vi "fields format list items from post.vi"(5 "Post (empty)":T1) -> (2 "List Options":string[](array[string]))   [LabVIEW 2011]
uses:
  Addons/internet/utils/keyedarr.llb/Keyed Array.ctl
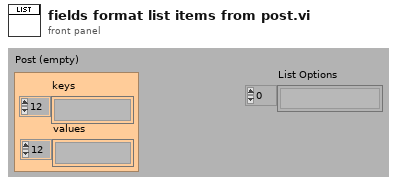
[diagram p1: front panel]
types:
  T1 = typedef "Keyed Array.ctl" = cluster{"keys":string[], "values":string[]}
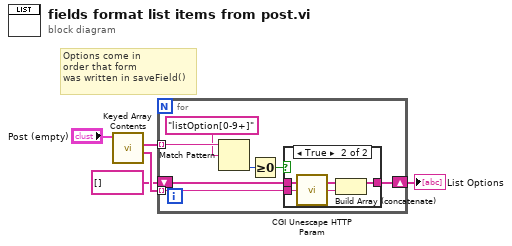
[diagram p0: block diagram]
diagram:
  # "Options come in\norder that form\nwas written in saveField()"
  n1 = call "Keyed Array Contents.vi"("array in"="Post (empty)") -> ("values"=w3:string[], "keys"=w4:string[])  [unwired: 5 out]
  n2 = for {
    tunnel: w4 -> [w12] mode=indexing
    tunnel: w3 -> [w9] mode=indexing
    shift-right: [w6] -> w1
    shift-left: string[] [] -> [w7]
    n3 = Match Pattern(string=w12, regular expression="listOption[0-9+]") -> (offset past match=w11:i32)  [unwired: 4 out]
    n4 = Greater Or Equal To 0?(x=w11) -> (x >= 0?=w8:bool)
    n5 = case shown="True" w8 {
      tunnel: w9 -> [_ w15]
      tunnel: w7 -> [w13 w17]
      tunnel: [w13 w16] -> w6
      frame False {
      }
      frame True {
        n6 = call "CGI Unescape HTTP Param.vi"("url-encoded string"=w15) -> ("string"=w14:string)
        n7 = Build Array (concatenate)(w17, w14) -> (w16:string[])
      }
    }
  }
  "List Options" <- w1
